vi "Matrix To Array - CM.vi"(1 "Complex Matrix":T1) -> (0 "Complex 2D Array":cdb[][](array[numeric]))   [LabVIEW 2018, in "NI_Matrix.lvlib"]
doc: "Converts a matrix of elements to an array of elements of the same data type. Wire data to the <B>Real Matrix</B> input to determine the polymorphic instance to use or manually select the instance."
uses:
  NI_Matrix.lvlib
  ComplexMatrix.ctl
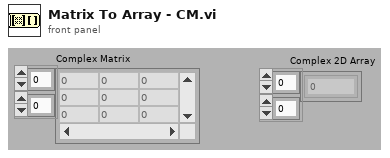
[diagram p1: front panel]
types:
  T1 = typedef "NI_Matrix.lvlib/ComplexMatrix.ctl" = cdb[][]
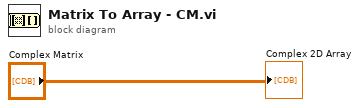
[diagram p0: block diagram]
diagram:
  "Complex 2D Array" <- "Complex Matrix"
